vi "SRV_PM_Trim Front of Unknown Packet Data.vi"(7 "1D Array":u8[](array[numeric])=[255, 255, 254, 255, 255, 255] format="%.0x", 9 "Search":u8[](array[numeric])=[255, 255, 255, 255] format="%.0x", 11 "error in (no error)":errorcluster) -> (8 "Trimmed 1D Array":u8[](array[numeric]) format="%.0x", 15 "error out":errorcluster)   [LabVIEW 2009]
doc: "Trimmed 1D Array is an array out that either begins with Search array or some portion of Search array that is potential to be Search array if more elements were added later or is empty if no instance of Search array or potential is found."
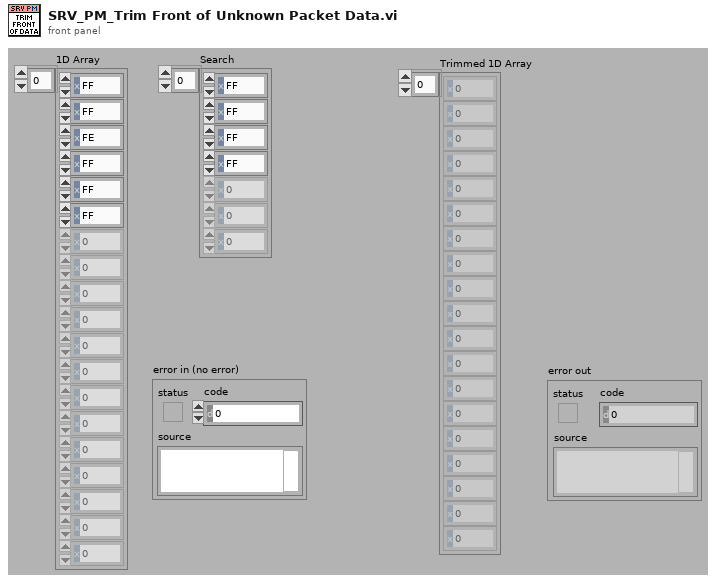
[diagram p1: front panel]
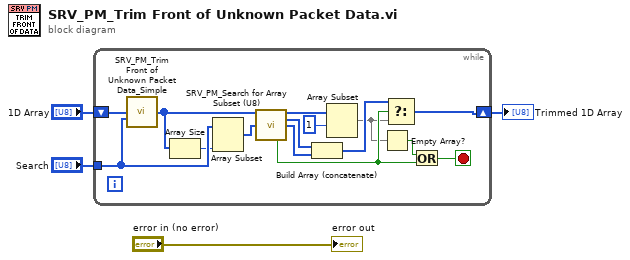
[diagram p0: block diagram]
diagram:
  n1 = while {
    shift-right: [w10] -> w2
    shift-left: "1D Array" -> [w19]
    tunnel: "Search" -> [w18]
    stop <- w5 stop-if-true
    n2 = call "SRV_PM_Trim Front of Unknown Packet Data_Simple.vi"("1D Array"=w19, "Search"=w18) -> ("Trimmed 1D Array"=w15:u8[])  [unwired: 13 in]
    n3 = Array Size(array=w15) -> (size(s)=w17:i32)
    n4 = Array Subset(array=w18, length=w17) -> (w16:u8[])  [unwired: 1 in]
    n5 = call "SRV_PM_Search for Array Subset (U8).vi"("1D Array"=w15, "Search"=w16) -> ("Before Match"=w9:u8[], "Match"=w14:u8[], "After Match"=w13:u8[], "Found?"=w11:bool)  [unwired: 8 in, 2 out]
    n6 = Build Array (concatenate)(w14, w13) -> (w12:u8[])
    n7 = Array Subset(array=w9, index=1) -> (w7:u8[])  [unwired: 1 in]
    n8 = Empty Array?(array=w7) -> (empty?=w6:bool)
    n9 = Select(t=w12, s=w11, f=w7) -> (s? t:f=w10:u8[])
    n10 = Or(x=w6, y=w11) -> (x .or. y?=w5:bool)
  }
  "Trimmed 1D Array" <- w2
  "error out" <- "error in (no error)"
